vi "list.vi"(8 "error in (no error)":errorcluster, 9 "parent node":string, 10 "tree reference":refnum<vi>, 11 "Map in":refnum<class "Map.lvclass">) -> (0 "error out":errorcluster)   [LabVIEW 2010, in "Map.lvclass"]
doc: "Lists the key-value entries in the map (a list for a non-nested map, or a tree for a nested map, respectively)."
uses:
  Map.lvclass
  Map.lvclass/Map.ctl
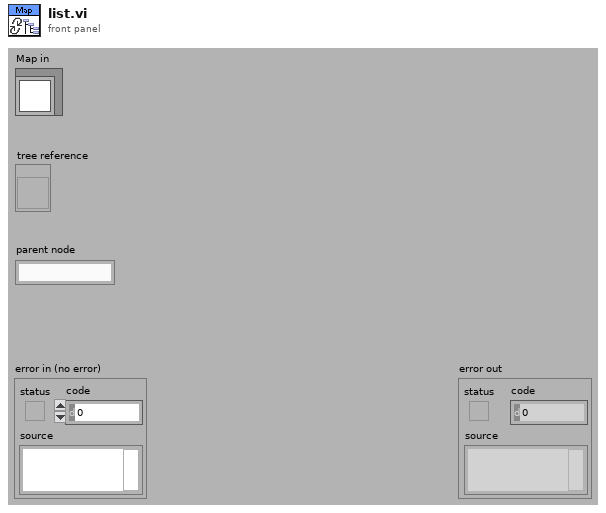
[diagram p1: front panel]
types:
  T1 = typedef "Map.lvclass/element_cluster.ctl" = cluster{"key":string, "value":variant}
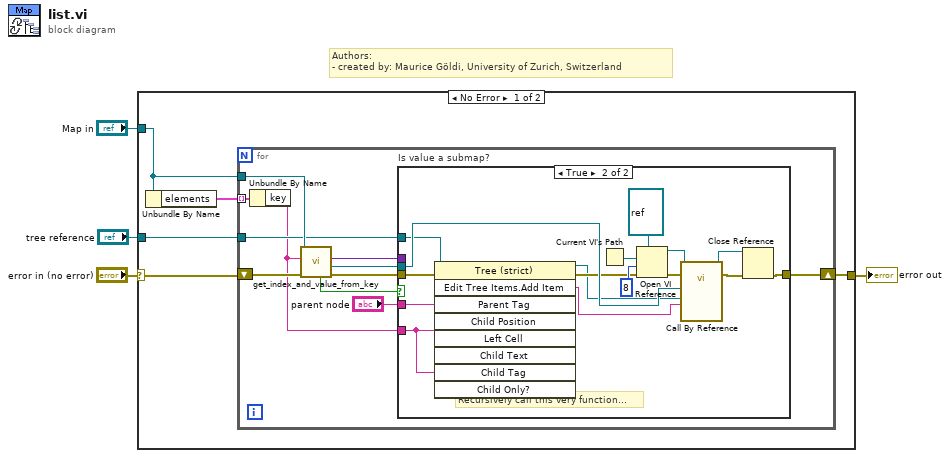
[diagram p0: block diagram]
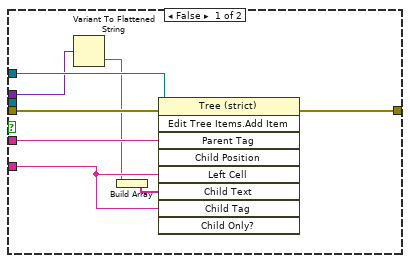
[diagram p2: hidden frame]
diagram:
  # "Authors: \n- created by: Maurice Göldi, University of Zurich, Switzerland"
  n1 = case shown="No Error" "error in (no error)" {
    selector: "error in (no error)" -> [w8 w45]
    tunnel: [w9 w45] -> w3
    tunnel: "Map in" -> [w6 _]
    tunnel: "tree reference" -> [w7 _]
    frame No Error {
      n2 = Unbundle By Name(w6) -> ("elements"=w5:T1[])
      n3 = for {
        shift-right: [w18] -> w9
        shift-left: w8 -> [w20]
        tunnel: w7 -> [w17]
        tunnel: w6 -> [w19]
        tunnel: w5 -> [w13] mode=indexing
        n4 = Unbundle By Name(w13) -> ("key"=w12:string)
        n5 = call "get_index_and_value_from_key.vi"("error in (no error)"=w20, "key"=w12, "Map.lvclass in"=w19) -> ("error out"=w14:errorcluster, "submap"=w15:refnum<class "Map.lvclass">, "value"=w16:variant, "submap?"=w10:bool)  [unwired: 5 out]
        n6 = case "Is value a submap?" shown="True" w10 {
          tunnel: w14 -> [w23 w34]
          tunnel: [w28 w37] -> w18
          tunnel: w17 -> [w27 w33]
          tunnel: w16 -> [w22 _]
          tunnel: w15 -> [_ w44]
          tunnel: w12 -> [w25 w30]
          tunnel: "parent node" -> [w24 w31]
          frame False {
            n7 = Variant To Flattened String(Variant=w22) -> (data string=w21:string)  [unwired: 1 out]
            n8 = Build Array(w21) -> (w26:string[])
            n9 = invoke class="Tree (strict)" method="Edit Tree Items.Add Item"(reference=w27, error in=w23, "Parent Tag"=w24, "Left Cell"=w25, "Child Text"=w26, "Child Tag"=w25) -> (error out=w28:errorcluster)  [unwired: 3 in, 8 out]
          }
          frame True {
            # "Recursively call this very function..."
            n10 = invoke class="Tree (strict)" method="Edit Tree Items.Add Item"(reference=w33, error in=w34, "Parent Tag"=w31, "Left Cell"=w30, "Child Tag"=w30) -> (reference out=w35:refnum<vi>, error out=w41:errorcluster, "Edit Tree Items:Add Item"=w29:string)  [unwired: 4 in, 6 out]
            n11 = Current VI's Path() -> (path=w42:path)
            n12 = Open VI Reference(type specifier VI Refnum (for type only)=refnum<vi> refnum, vi path=w42, options=8, error in (no error)=w41) -> (vi reference=w39:refnum<vi>, error out=w40:errorcluster)  [unwired: 2 out]
            n13 = call-by-ref "?"(reference=w39, error in=w40, "parent node"=w29, "tree reference"=w35, "Map in"=w44) -> (reference out=w36:refnum<vi>, error out=w38:errorcluster)  [unwired: 8 in, 1 out]
            n14 = Close Reference(reference=w36, error in (no error)=w38) -> (error out=w37:errorcluster)
          }
        }
      }
    }
    frame Error {
    }
  }
  "error out" <- w3
